vi "stage_move.vi"(1 "Delay Cluster":T1={"System no."=0, "Identification"="", "Device ID out"=0, "Postion / mm"=[], "SN out"="", "Movement Range"=[], "Conn. Axes"=[], "Target Position / mm"=50.0, "Velocity / mm s^-1"=0.15, "Current Pos"=0.0, "Set-up"=FALSE, "Moving"=FALSE, "Step Size / mm "=0.15}, 3 "No.of digits":i16=4, 4 "Gap":dbl=0.5, 6 "Stop ref":refnum<vi>, 7 "stage_num":i32, 9 "position ref":refnum<vi>, 11 "Stage error in":errorcluster, 14 "polling time":u32=100) -> (8 "Final position":dbl, 10 "Direction":bool, 15 "Stage error out":errorcluster)   [LabVIEW 2015]
doc: "This vi will move the stage to the desitination, AND the stage approachs the destination from defined direction depending the direction-flag. Step determines the overshoot distance.\nAfter this, the velocity is set to final velocity for further small step measurements."
uses:
  Type defs/PI_delay_settings.ctl
  <vilib>/Utility/error.llb/DialogType.ctl
panel:
  out "Position":dbl[](array[numeric]) format="%.6f"
  in  "stop":bool
  in  "Final Velocity":dbl=1.5
  in  "Moving Velocity":dbl=1.5
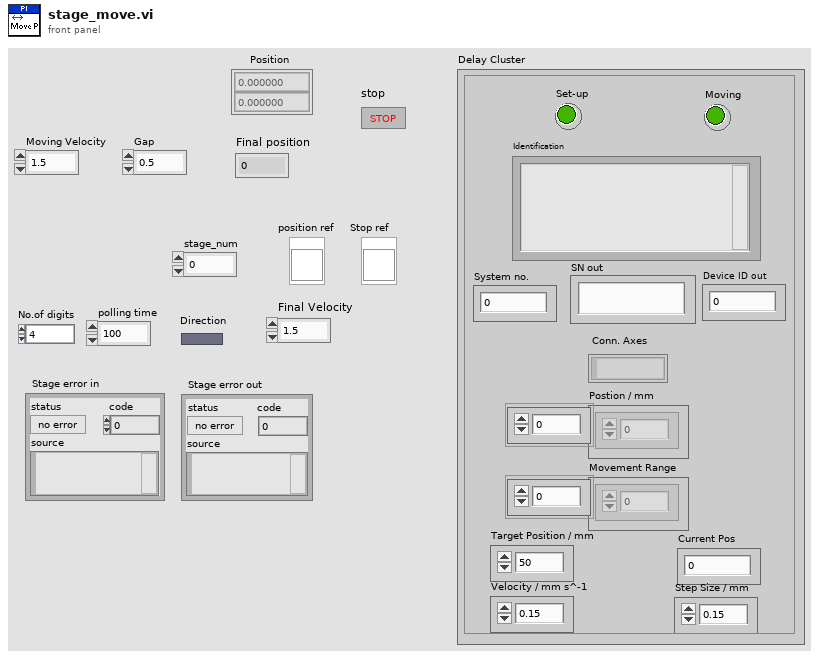
[diagram p1: front panel]
types:
  T1 = typedef "PI_delay_settings.ctl" = cluster{"System no.":i32, "Identification":string, "Device ID out":i32, "Postion / mm":dbl[], "SN out":string, "Movement Range":dbl[], "Conn. Axes":string[], "Target Position / mm":dbl, "Velocity / mm s^-1":dbl, "Current Pos":dbl, "Set-up":bool, "Moving":bool, "Step Size / mm ":dbl}
  T2 = typedef "DialogType.ctl" = u16
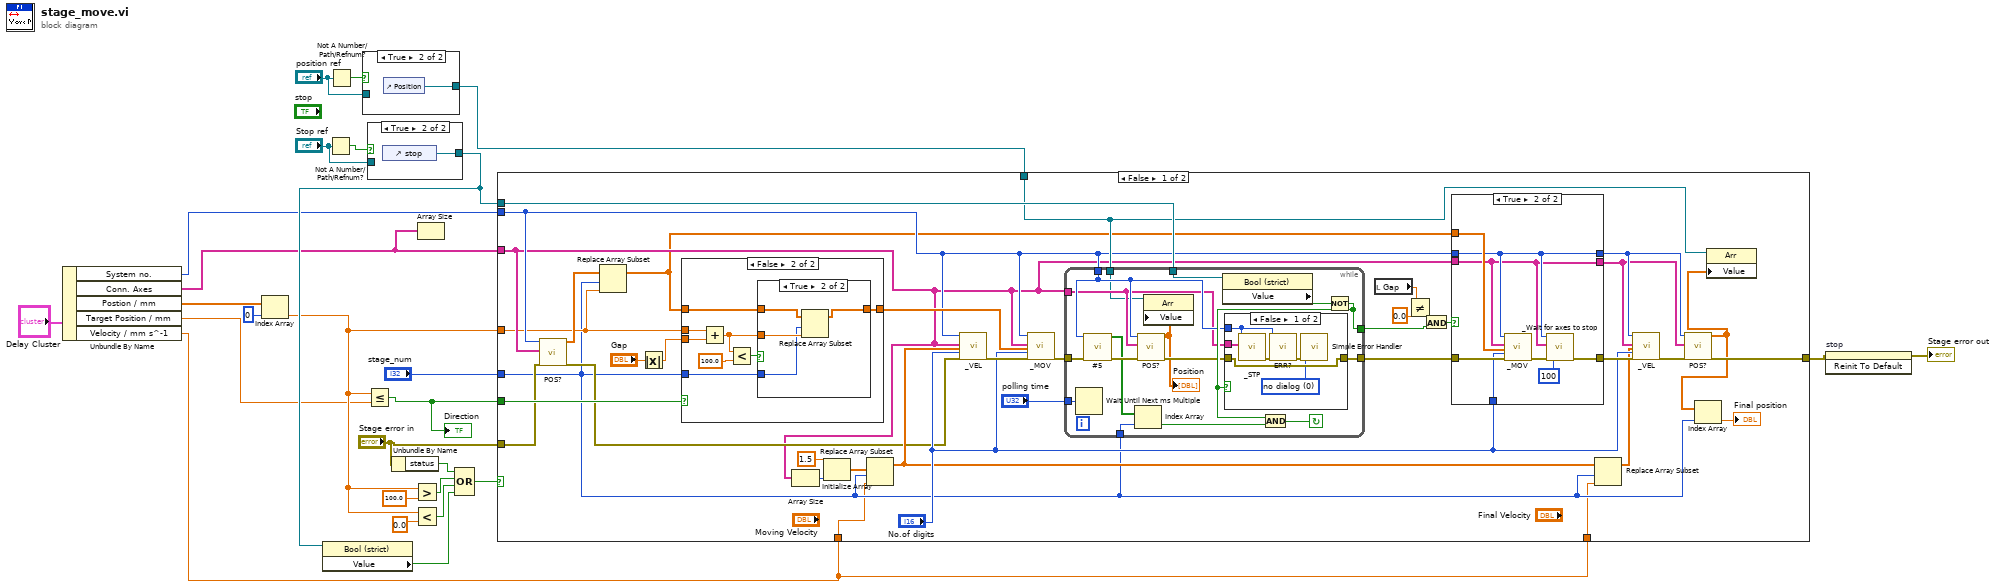
[diagram p0: block diagram]
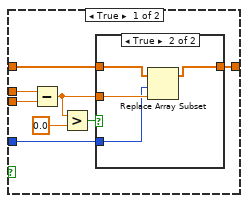
[diagram p6: hidden frame]
diagram:
  n1 = Unbundle By Name("Delay Cluster") -> ("System no."=w7:i32, "Conn. Axes"=w6:string[], "Postion / mm"=w5:dbl[], "Target Position / mm"=w2:dbl, "Velocity / mm s^-1"=w1:dbl)
  n2 = Index Array(array=w5, index=0) -> (element=w3:dbl)
  n3 = Not A Number/Path/Refnum?(number/path/refnum="Stop ref") -> (NaN/Path/Refnum?=w17:bool)
  n4 = Not A Number/Path/Refnum?(number/path/refnum="position ref") -> (NaN/Path/Refnum?=w13:bool)
  n5 = case shown="True" w13 {
    tunnel: [w27 w28] -> w9
    tunnel: "position ref" -> [w27 _]
    frame False {
    }
    frame True {
      n6 = control-ref of="Position"() -> (w28:refnum<vi>)
    }
  }
  n7 = Less Or Equal?(x=w3, y=w2) -> (x <= y?=w18:bool)
  "Direction" <- w18
  n8 = case shown="True" w17 {
    tunnel: [w29 w30] -> w15
    tunnel: "Stop ref" -> [w29 _]
    frame False {
    }
    frame True {
      n9 = control-ref of="stop"() -> (w30:refnum<vi>)
    }
  }
  n10 = property class="Bool (strict)"(reference=w15) -> ("Value"=w14:bool)  [unwired: 1 in, 2 out]
  n11 = Unbundle By Name("Stage error in") -> ("status"=w24:bool)
  n12 = Greater?(x=w3, y=100.0) -> (0:w22:bool)
  n13 = Less?(x=w3, y=0.0) -> (x < y?=w21:bool)
  n14 = Array Size(array=w6) -> ()  [unwired: 1 out]
  n15 = Compound Arithmetic op=OR(w24, w22, w21, w14) -> (w23:bool)
  n16 = case shown="False" w23 {
    tunnel: [w47 w129] -> w11
    tunnel: "stage_num" -> [w34 _]
    tunnel: w3 -> [w35 _]
    tunnel: "Stage error in" -> [w40 w129]
    tunnel: w6 -> [w37 _]
    tunnel: w18 -> [w55 _]
    tunnel: w15 -> [w54 _]
    tunnel: w9 -> [w44 _]
    tunnel: w7 -> [w38 _]
    tunnel: w1 -> [w32 _]
    tunnel: w1 -> [w31 _]
    frame False {
      n17 = call "POS?.vi"("System no."=w38, "Axes to query"=w37, "error in"=w40) -> ("Position"=w36:dbl[], "error out"=w39:errorcluster)  [unwired: 15 in]
      n18 = Replace Array Subset(array=w36, new element=w35, index=w34) -> (w33:dbl[])
      n19 = Absolute Value(x="Gap") -> (abs(x)=w67:dbl)
      n20 = case shown="False" w55 {
        tunnel: w35 -> [w110 w123]
        tunnel: w34 -> [w106 w119]
        tunnel: w33 -> [w105 w118]
        tunnel: [w104 w117] -> w63
        tunnel: w67 -> [w103 w116]
        frame True {
          n21 = Subtract(x=w110, y=w103) -> (x-y=w107:dbl)
          n22 = Greater?(x=w107, y=0.0) -> (0:w109:bool)
          n23 = case shown="True" w109 {
            tunnel: w107 -> [_ w115]
            tunnel: w106 -> [_ w114]
            tunnel: w105 -> [w111 w113]
            tunnel: [w111 w112] -> w104
            frame False {
            }
            frame True {
              n24 = Replace Array Subset(array=w113, new element=w115, index=w114) -> (w112:dbl[])
            }
          }
        }
        frame False {
          n25 = Add(x=w123, y=w116) -> (x+y=w120:dbl)
          n26 = Less?(x=w120, y=100.0) -> (x < y?=w122:bool)
          n27 = case shown="True" w122 {
            tunnel: w120 -> [_ w128]
            tunnel: w119 -> [_ w127]
            tunnel: w118 -> [w124 w126]
            tunnel: [w124 w125] -> w117
            frame False {
            }
            frame True {
              n28 = Replace Array Subset(array=w126, new element=w128, index=w127) -> (w125:dbl[])
            }
          }
        }
      }
      n29 = Array Size(array=w37) -> (size(s)=w62:i32)
      n30 = Initialize Array(1.5 ("element"), w62) -> (w60:dbl[])
      n31 = Replace Array Subset(array=w60, new element=w32, index=w34) -> (w57:dbl[])
      n32 = call "_VEL.vi"("System no."=w38, "Axes to set"=w37, "Velocity values"=w57, "No.of digits"="No.of digits", "error in"=w39) -> ("error out"=w66:errorcluster)  [unwired: 13 in, 1 out]
      n33 = call "_MOV.vi"("System no."=w38, "Axes to move"=w37, "Position values"=w63, "No.of digits"="No.of digits", "error in"=w66) -> ("error out"=w65:errorcluster)  [unwired: 14 in]
      n34 = while {
        tunnel: w65 -> [w87]
        tunnel: "polling time" -> [w95]
        tunnel: w38 -> [w83]
        tunnel: w37 -> [w82]
        tunnel: [w89] -> w41
        tunnel: w44 -> [w81]
        tunnel: w34 -> [w94]
        tunnel: w54 -> [w93]
        tunnel: [w88] -> w49
        stop <- w91 continue-if-true
        n35 = Wait Until Next ms Multiple(millisecond multiple=w95) -> ()  [unwired: 1 out]
        n36 = call "#5.vi"("System no."=w83, "error in"=w87) -> ("Axis moving?"=w84:bool[], "error out"=w86:errorcluster)  [unwired: 16 in]
        n37 = Index Array(array=w84, index=w94) -> (element=w92:bool)
        n38 = call "POS?.vi"("System no."=w83, "Axes to query"=w82, "error in"=w86) -> ("Position"=w80:dbl[], "error out"=w85:errorcluster)  [unwired: 15 in]
        "Position" <- w80
        n39 = property class="Arr"(reference=w81, "Value"=w80) -> ()  [unwired: 1 in, 2 out]
        n40 = property class="Bool (strict)"(reference=w93) -> ("Value"=w90:bool)  [unwired: 1 in, 2 out]
        n41 = Not(x=w90) -> (.not. x?=w88:bool)
        n42 = case shown="False" w88 {
          tunnel: [w98 w102] -> w89
          tunnel: w85 -> [w98 w102]
          tunnel: w83 -> [w99 _]
          tunnel: w82 -> [w101 _]
          frame False {
            w96 = T2 0 items=["no dialog", "OK message", "continue or stop message", "OK message + warnings", "continue/stop + warnings"] ("type of dialog (OK msg:1)")
            n43 = call "_STP.vi"("System no."=w99, "Affected axes?"=w101) -> ("error out"=w100:errorcluster)  [unwired: 17 in]
            n44 = call "ERR?.vi"("System no."=w99, "error in"=w100) -> ("error out"=w97:errorcluster)  [unwired: 16 in, 1 out]
            n45 = call <vilib>:"Simple Error Handler.vi"("type of dialog (OK msg:1)"=w96, "error in (no error)"=w97) -> ()  [unwired: 3 in, 5 out]
          }
          frame True {
          }
        }
        n46 = And(x=w88, y=w92) -> (x .and. y?=w91:bool)
      }
      n47 = local read "Gap"() -> (w53:dbl)
      n48 = Not Equal?(x=w53, y=0.0) -> (x != y?=w51:bool)
      n49 = And(x=w51, y=w49) -> (x .and. y?=w50:bool)
      n50 = case shown="True" w50 {
        tunnel: w41 -> [w71 w79]
        tunnel: w33 -> [_ w78]
        tunnel: [w71 w74] -> w59
        tunnel: "No.of digits" -> [_ w77]
        tunnel: w38 -> [w70 w73]
        tunnel: w37 -> [w69 w72]
        tunnel: [w70 w73] -> w43
        tunnel: [w69 w72] -> w42
        frame False {
        }
        frame True {
          n51 = call "_MOV.vi"("System no."=w73, "Axes to move"=w72, "Position values"=w78, "No.of digits"=w77, "error in"=w79) -> ("error out"=w76:errorcluster)  [unwired: 14 in]
          n52 = call "_Wait for axes to stop.vi"("System no."=w73, "Axes to wait for"=w72, "error in"=w76, "Polling cycle time, ms"=u32 100) -> ("error out"=w74:errorcluster)  [unwired: 14 in, 1 out]
        }
      }
      n53 = Replace Array Subset(array=w57, new element=w31, index=w34) -> (w56:dbl[])
      n54 = call "_VEL.vi"("System no."=w43, "Axes to set"=w42, "Velocity values"=w56, "No.of digits"="No.of digits", "error in"=w59) -> ("error out"=w48:errorcluster)  [unwired: 13 in, 1 out]
      n55 = call "POS?.vi"("System no."=w43, "Axes to query"=w42, "error in"=w48) -> ("Position"=w45:dbl[], "error out"=w47:errorcluster)  [unwired: 15 in]
      n56 = Index Array(array=w45, index=w34) -> (element=→"Final position":dbl)
      n57 = property class="Arr"(reference=w44, "Value"=w45) -> ()  [unwired: 1 in, 2 out]
    }
    frame True {
    }
  }
  n58 = invoke on="stop" class="Bool (strict)" method="Reinit To Default"(error in=w11) -> (error out=→"Stage error out":errorcluster)  [unwired: 2 in, 2 out]
